vi "hpcnc hack autorun.vi"(7 "error in (no error)":errorcluster, 9 "Idle":bool, 10 "VISA Refnum in":refnum<visa-resource-name>) -> (1 "Reset":bool)   [LabVIEW 2014]
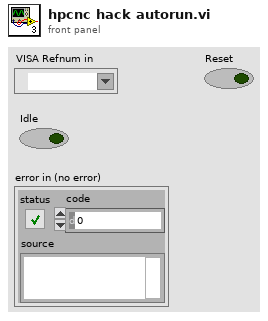
[diagram p1: front panel]
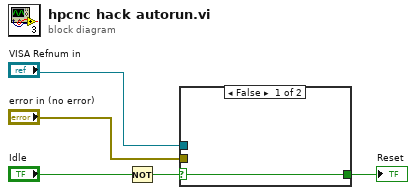
[diagram p0: block diagram]
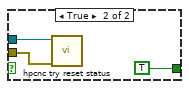
[diagram p2: hidden frame]
diagram:
  n1 = Not(x="Idle") -> (.not. x?=w2:bool)
  n2 = case shown="False" w2 {
    selector: w2 -> [w6 _]
    tunnel: [w6 TRUE] -> w3
    tunnel: "VISA Refnum in" -> [_ w9]
    tunnel: "error in (no error)" -> [_ w7]
    frame False {
    }
    frame True {
      n3 = call "hpcnc try reset status.vi"("error in (no error)"=w7, "VISA Refnum in"=w9) -> ()  [unwired: 10 in]
    }
  }
  "Reset" <- w3
